vi "Demo_3 - Channel device_Main .vi"() -> ()   [LabVIEW 2011]
uses:
  <instrlib>/Thorlabs_MDT69xB/Thorlabs_MDT69xB.lvlib
panel:
  in  "Set Master Scan Enable?":bool
  out "Get MS Voltage(V)":dbl
  in  "Set MS Voltage(V)":dbl
  out "Get z Voltage(V)":dbl
  out "Get y Voltage(V)":dbl
  out "Get x Voltage(V)":dbl
  in  "Set z Voltage(V)":dbl
  in  "Set y Voltage(V)":dbl
  in  "Set x Voltage(V)":dbl
  out "Master Scan Enable?":bool
  out "v limit(V)":dbl
  out "?":string
  # "Device Info"
  # "Set Params"
  # "Get Params"
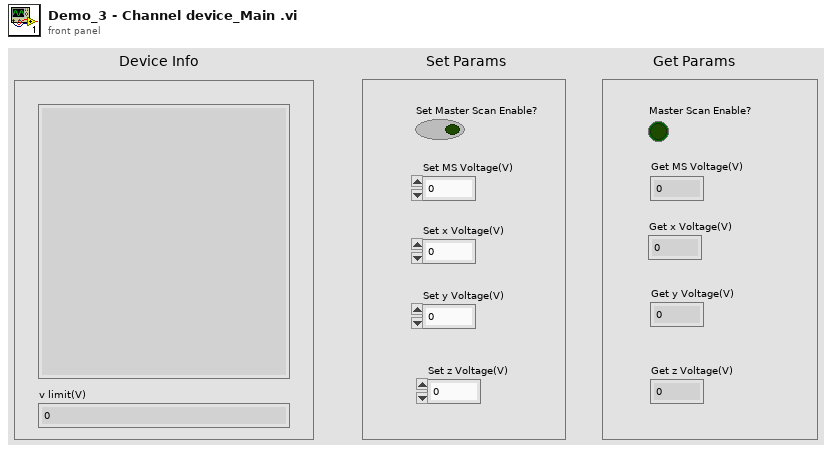
[diagram p1: front panel]
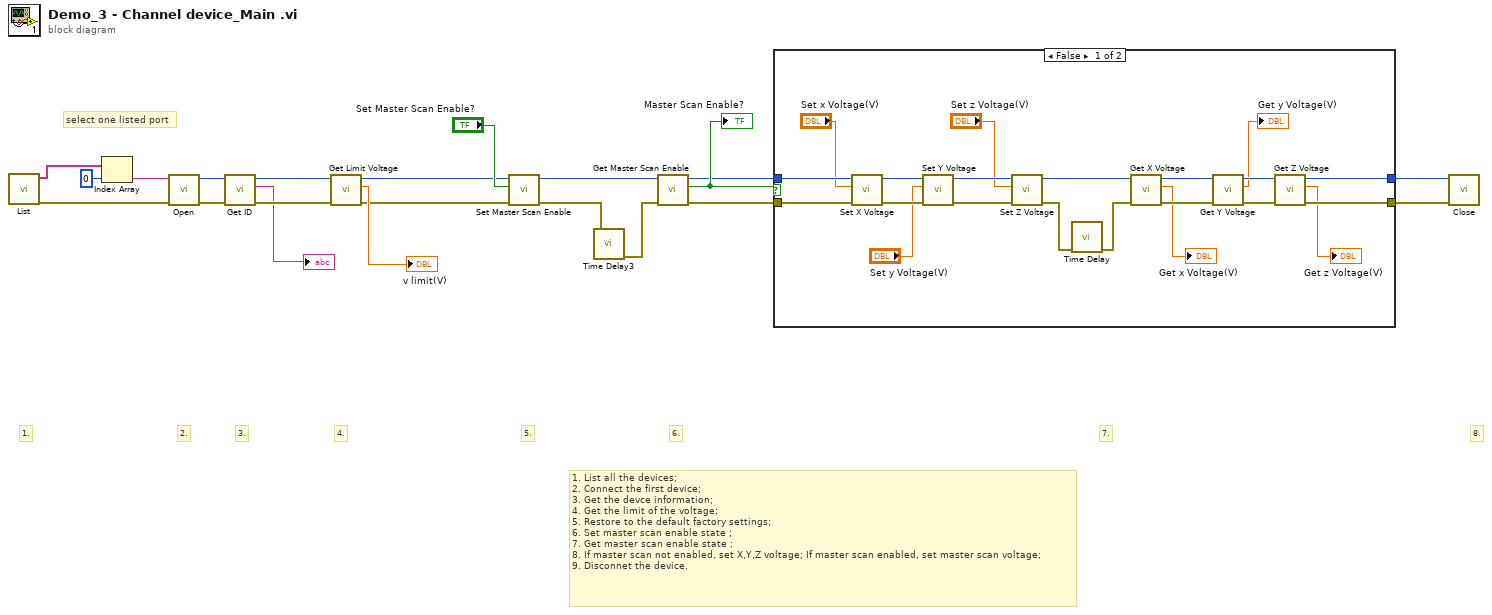
[diagram p0: block diagram]
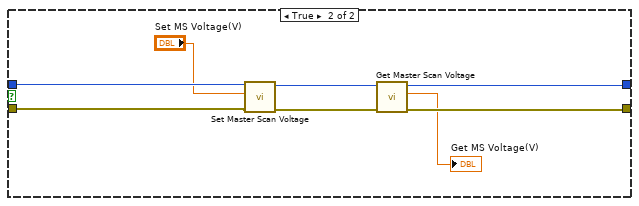
[diagram p2: hidden frame]
diagram:
  # "8."
  # "7."
  # "6."
  # "5."
  # "1. List all the devices;\n2. Connect the first device;\n3. Get the devce information;\n4. Get the limit of the voltage;\n5. Restore to the default factory settings;\n6. Set master scan enable state ;\n7. Get master scan enable state ;\n8. If master scan not enabled, set X,Y,Z voltage; If master scan enabled, set master scan voltage; \n9. Disconnet the device."
  # "4."
  # "3."
  # "2."
  # "1."
  # "select one listed port"
  n1 = call <instrlib>:"List.vi"() -> ("error out"=w18:errorcluster, "COM ports"=w21:string[])  [unwired: 10 in]
  n2 = Index Array(array=w21, index=0) -> (element=w19:string)
  n3 = call <instrlib>:"Open.vi"("error in (no error)"=w18, "Serial Port"=w19) -> ("error out"=w17:errorcluster, "hDevice"=w16:i32)  [unwired: 7 in, 1 out]
  n4 = call <instrlib>:"Get ID.vi"("error in (no error)"=w17, "hdl in"=w16) -> ("error out"=w14:errorcluster, "ID"=→"?":string, "hdl out"=w15:i32)  [unwired: 7 in]
  n5 = call <instrlib>:"Get Limit Voltage.vi"("error in (no error)"=w14, "hdl in"=w15) -> ("error out"=w2:errorcluster, "v limit"=→"v limit(V)":dbl, "hdl out"=w3:i32)  [unwired: 7 in]
  n6 = call <instrlib>:"Set Master Scan Enable.vi"("error in (no error)"=w2, "Set Master Scan Enable?"="Set Master Scan Enable?", "hdl in"=w3) -> ("error out"=w5:errorcluster, "hdl"=w11:i32)  [unwired: 7 in]
  n7 = call "Time Delay3"("error in (no error)"=w5) -> ("error out"=w10:errorcluster)  [unwired: 10 in]
  n8 = call <instrlib>:"Get Master Scan Enable.vi"("error in (no error)"=w10, "hdl in"=w11) -> ("error out"=w7:errorcluster, "Master Scan Enable?"=w9:bool, "hdl out"=w8:i32)  [unwired: 7 in]
  "Master Scan Enable?" <- w9
  n9 = case shown="False" w9 {
    tunnel: w8 -> [w42 w50]
    tunnel: w7 -> [w40 w47]
    tunnel: [w30 w48] -> w6
    tunnel: [w29 w45] -> w1
    frame False {
      n10 = call <instrlib>:"Set X Voltage.vi"("error in (no error)"=w40, "Set x Voltage(V)"="Set x Voltage(V)", "hdl in"=w42) -> ("error out"=w39:errorcluster, "hdl"=w41:i32)  [unwired: 7 in]
      n11 = call <instrlib>:"Set Y Voltage.vi"("error in (no error)"=w39, "Set y Voltage(V)"="Set y Voltage(V)", "hdl in"=w41) -> ("error out"=w38:errorcluster, "hdl"=w37:i32)  [unwired: 7 in]
      n12 = call <instrlib>:"Set Z Voltage.vi"("error in (no error)"=w38, "Set z Voltage(V)"="Set z Voltage(V)", "hdl in"=w37) -> ("error out"=w35:errorcluster, "hdl"=w36:i32)  [unwired: 7 in]
      n13 = call "Time Delay"("error in (no error)"=w35) -> ("error out"=w22:errorcluster)  [unwired: 10 in]
      n14 = call <instrlib>:"Get X Voltage.vi"("error in (no error)"=w22, "hdl in"=w36) -> ("error out"=w33:errorcluster, "Get x Voltage(V)"=→"Get x Voltage(V)":dbl, "hdl"=w34:i32)  [unwired: 7 in]
      n15 = call <instrlib>:"Get Y Voltage.vi"("error in (no error)"=w33, "hdl in"=w34) -> ("error out"=w31:errorcluster, "Get y Voltage(V)"=→"Get y Voltage(V)":dbl, "hdl"=w32:i32)  [unwired: 7 in]
      n16 = call <instrlib>:"Get Z Voltage.vi"("error in (no error)"=w31, "hdl in"=w32) -> ("error out"=w29:errorcluster, "Get z Voltage(V)"=→"Get z Voltage(V)":dbl, "hdl"=w30:i32)  [unwired: 7 in]
    }
    frame True {
      n17 = call <instrlib>:"Set Master Scan Voltage.vi"("error in (no error)"=w47, "Set MS Voltage(V)"="Set MS Voltage(V)", "hdl in"=w50) -> ("error out"=w46:errorcluster, "hdl"=w49:i32)  [unwired: 7 in]
      n18 = call <instrlib>:"Get Master Scan Voltage.vi"("error in (no error)"=w46, "hdl in"=w49) -> ("error out"=w45:errorcluster, "Get MS Voltage(V)"=→"Get MS Voltage(V)":dbl, "hdl"=w48:i32)  [unwired: 7 in]
    }
  }
  n19 = call <instrlib>:"Close.vi"("error in (no error)"=w1, "hDevice"=w6) -> ()  [unwired: 9 in, 1 out]
